vi "3001-CC.VI"() -> ()   [LabVIEW 2015]
uses:
  board.vis/Globals.vi
  <vilib>/Analysis/NI_AALBase.lvlib
panel:
  out "CAMCNT":dbl=2.0
  in  "extTrig":bool
  in  "ext. trig. slope":enum32{"1", "2", "3"}(radio)
  out "amount of devices":u8=1
  out "amount of cams":u8=2
  in  "CHB 8":bool
  in  "CHA 8":bool
  in  "CHB 7":bool
  in  "CHA 7":bool
  in  "CHB 6":bool
  in  "CHA 6":bool
  in  "CHB 5":bool
  in  "CHA 5":bool
  in  "CHB 4":bool
  in  "CHA 4":bool
  in  "CHB 3":bool
  in  "CHA 3":bool
  in  "CHB 2":bool
  in  "CHA 2":bool
  in  "CHB 1":bool=TRUE
  in  "CHA 1":bool=TRUE
  in  "channel quick select (in hex)":u16=3 format="%x"
  out "tRMS":dbl format="%0#.1f"
  out "mean":dbl format="%#_4f"
  in  "rms_pixel":u16=100
  in  "is FFT":bool=TRUE
  in  "IR gain":bool
  in  "continuous":bool=TRUE
  out "curr.block":u8=2
  out "Measure ON":bool
  in  "Board select\n1: board 1\n2: board 2\n3: both boards":u8=3
  in  "no.of blocks (nob)\npress enter":u32=1
  in  "block":u32(slide)=1 max=10 scale=0.9..1.0
  out "Signalverlaufgraph 2":u16[](graph)=[0, 0, 543, 543, 0, 1, 0, 0, 2, 2, 3, 3, 4, 4, 5, 5, 6, 6, 7, 7, 8, 8, 9, 9, 10, 10, 11, 11, 12, 12, 13, 13, 14, 14, 15, 15, 16, 16, 17, 17, 18, 18, 19, 19, 20, 20, 21, 21, 22, 22, 23, 23, 24, 24, 25, 25, 26, 26, 27, 27, 28, 28, 29, 29, 30, 30, 31, 31, 32, 32, 33, 33, 34, 34, 35, 35, 36, 36, 37, 37, 38, 38, 39, 39, 40, 40, 41, 41, 42, 42, 43, 43, 44, 44, 45, 45, 46, 46, 47, 47, 48, 48, 49, 49, 50, 50, 51, 51, 52, 52, 53, 53, 54, 54, 55, 55, 56, 56, 57, 57, 58, 58, 59, 59, 60, 60, 61, 61, 62, 62, 63, 63, 64, 64, 65, 65, 66, 66, 67, 67, 68, 68, 69, 69, 70, 70, 71, 71, 72, 72, 73, 73, 74, 74, 75, 75, 76, 76, 77, 77, 78, 78, 79, 79, 80, 80, 81, 81, 82, 82, 83, 83, 84, 84, 85, 85, 86, 86, 87, 87, 88, 88, 89, 89, 90, 90, 91, 91, 92, 92, 93, 93, 94, 94, 95, 95, 96, 96, 97, 97, 98, 98, 99, 99, 100, 100, 101, 101, 102, 102, 103, 103, 104, 104, 105, 105, 106, 106, 107, 107, 108, 108, 109, 109, 110, 110, 111, 111, 112, 112, 113, 113, 114, 114, 115, 115, 116, 116, 117, 117, 118, 118, 119, 119, 120, 120, 121, 121, 122, 122, 123, 123, 124, 124, 125, 125, 126, 126, 127, 127, 128, 128, 129, 129, 130, 130, 131, 131, 132, 132, 133, 133, 134, 134, 135, 135, 136, 136, 137, 137, 138, 138, 139, 139, 140, 140, 141, 141, 142, 142, 143, 143, 144, 144, 145, 145, 146, 146, 147, 147, 148, 148, 149, 149, 150, 150, 151, 151, 152, 152, 153, 153, 154, 154, 155, 155, 156, 156, 157, 157, 158, 158, 159, 159, 160, 160, 161, 161, 162, 162, 163, 163, 164, 164, 165, 165, 166, 166, 167, 167, 168, 168, 169, 169, 170, 170, 171, 171, 172, 172, 173, 173, 174, 174, 175, 175, 176, 176, 177, 177, 178, 178, 179, 179, 180, 180, 181, 181, 182, 182, 183, 183, 184, 184, 185, 185, 186, 186, 187, 187, 188, 188, 189, 189, 190, 190, 191, 191, 192, 192, 193, 193, 194, 194, 195, 195, 196, 196, 197, 197, 198, 198, 199, 199, 200, 200, 201, 201, 202, 202, 203, 203, 204, 204, 205, 205, 206, 206, 207, 207, 208, 208, 209, 209, 210, 210, 211, 211, 212, 212, 213, 213, 214, 214, 215, 215, 216, 216, 217, 217, 218, 218, 219, 219, 220, 220, 221, 221, 222, 222, 223, 223, 224, 224, 225, 225, 226, 226, 227, 227, 228, 228, 229, 229, 230, 230, 231, 231, 232, 232, 233, 233, 234, 234, 235, 235, 236, 236, 237, 237, 238, 238, 239, 239, 240, 240, 241, 241, 242, 242, 243, 243, 244, 244, 245, 245, 246, 246, 247, 247, 248, 248, 249, 249, 250, 250, 251, 251, 252, 252, 253, 253, 254, 254, 255, 255, 256, 256, 257, 257, 258, 258, 259, 259, 260, 260, 261, 261, 262, 262, 263, 263, 264, 264, 265, 265, 266, 266, 267, 267, 268, 268, 269, 269, 270, 270, 271, 271, 272, 272, 273, 273, 274, 274, 275, 275, 276, 276, 277, 277, 278, 278, 279, 279, 280, 280, 281, 281, 282, 282, 283, 283, 284, 284, 285, 285, 286, 286, 287, 287, 288, 288, 289, 289, 290, 290, 291, 291, 292, 292, 293, 293, 294, 294, 295, 295, 296, 296, 297, 297, 298, 298, 299, 299, 300, 300, 301, 301, 302, 302, 303, 303, 304, 304, 305, 305, 306, 306, 307, 307, 308, 308, 309, 309, 310, 310, 311, 311, 312, 312, 313, 313, 314, 314, 315, 315, 316, 316, 317, 317, 318, 318, 319, 319, 320, 320, 321, 321, 322, 322, 323, 323, 324, 324, 325, 325, 326, 326, 327, 327, 328, 328, 329, 329, 330, 330, 331, 331, 332, 332, 333, 333, 334, 334, 335, 335, 336, 336, 337, 337, 338, 338, 339, 339, 340, 340, 341, 341, 342, 342, 343, 343, 344, 344, 345, 345, 346, 346, 347, 347, 348, 348, 349, 349, 350, 350, 351, 351, 352, 352, 353, 353, 354, 354, 355, 355, 356, 356, 357, 357, 358, 358, 359, 359, 360, 360, 361, 361, 362, 362, 363, 363, 364, 364, 365, 365, 366, 366, 367, 367, 368, 368, 369, 369, 370, 370, 371, 371, 372, 372, 373, 373, 374, 374, 375, 375, 376, 376, 377, 377, 378, 378, 379, 379, 380, 380, 381, 381, 382, 382, 383, 383, 384, 384, 385, 385, 386, 386, 387, 387, 388, 388, 389, 389, 390, 390, 391, 391, 392, 392, 393, 393, 394, 394, 395, 395, 396, 396, 397, 397, 398, 398, 399, 399, 400, 400, 401, 401, 402, 402, 403, 403, 404, 404, 405, 405, 406, 406, 407, 407, 408, 408, 409, 409, 410, 410, 411, 411, 412, 412, 413, 413, 414, 414, 415, 415, 416, 416, 417, 417, 418, 418, 419, 419, 420, 420, 421, 421, 422, 422, 423, 423, 424, 424, 425, 425, 426, 426, 427, 427, 428, 428, 429, 429, 430, 430, 431, 431, 432, 432, 433, 433, 434, 434, 435, 435, 436, 436, 437, 437, 438, 438, 439, 439, 440, 440, 441, 441, 442, 442, 443, 443, 444, 444, 445, 445, 446, 446, 447, 447, 448, 448, 449, 449, 450, 450, 451, 451, 452, 452, 453, 453, 454, 454, 455, 455, 456, 456, 457, 457, 458, 458, 459, 459, 460, 460, 461, 461, 462, 462, 463, 463, 464, 464, 465, 465, 466, 466, 467, 467, 468, 468, 469, 469, 470, 470, 471, 471, 472, 472, 473, 473, 474, 474, 475, 475, 476, 476, 477, 477, 478, 478, 479, 479, 480, 480, 481, 481, 482, 482, 483, 483, 484, 484, 485, 485, 486, 486, 487, 487, 488, 488, 489, 489, 490, 490, 491, 491, 492, 492, 493, 493, 494, 494, 495, 495, 496, 496, 497, 497, 498, 498, 499, 499, 500, 500, 501, 501, 502, 502, 503, 503, 504, 504, 505, 505, 506, 506, 507, 507, 508, 508, 509, 509, 510, 510, 511, 511, 512, 512, 513, 513, 514, 514, 515, 515, 516, 516, 517, 517, 518, 518, 519, 519, 520, 520, 521, 521, 522, 522, 523, 523, 524, 524, 525, 525, 526, 526, 527, 527, 528, 528, 529, 529, 530, 530, 531, 531, 532, 532, 533, 533, 534, 534, 535, 535, 536, 536, 537, 537, 538, 538, 539, 539, 540, 540, 541, 541]
  out "Signalverlaufgraph":u16[](graph)=[544, 544, 545, 545, 49152, 1, 0, 0, 2, 2, 3, 3, 4, 4, 5, 5, 6, 6, 7, 7, 8, 8, 9, 9, 10, 10, 11, 11, 12, 12, 13, 13, 14, 14, 15, 15, 16, 16, 17, 17, 18, 18, 19, 19, 20, 20, 21, 21, 22, 22, 23, 23, 24, 24, 25, 25, 26, 26, 27, 27, 28, 28, 29, 29, 30, 30, 31, 31, 32, 32, 33, 33, 34, 34, 35, 35, 36, 36, 37, 37, 38, 38, 39, 39, 40, 40, 41, 41, 42, 42, 43, 43, 44, 44, 45, 45, 46, 46, 47, 47, 48, 48, 49, 49, 50, 50, 51, 51, 52, 52, 53, 53, 54, 54, 55, 55, 56, 56, 57, 57, 58, 58, 59, 59, 60, 60, 61, 61, 62, 62, 63, 63, 64, 64, 65, 65, 66, 66, 67, 67, 68, 68, 69, 69, 70, 70, 71, 71, 72, 72, 73, 73, 74, 74, 75, 75, 76, 76, 77, 77, 78, 78, 79, 79, 80, 80, 81, 81, 82, 82, 83, 83, 84, 84, 85, 85, 86, 86, 87, 87, 88, 88, 89, 89, 90, 90, 91, 91, 92, 92, 93, 93, 94, 94, 95, 95, 96, 96, 97, 97, 98, 98, 99, 99, 100, 100, 101, 101, 102, 102, 103, 103, 104, 104, 105, 105, 106, 106, 107, 107, 108, 108, 109, 109, 110, 110, 111, 111, 112, 112, 113, 113, 114, 114, 115, 115, 116, 116, 117, 117, 118, 118, 119, 119, 120, 120, 121, 121, 122, 122, 123, 123, 124, 124, 125, 125, 126, 126, 127, 127, 128, 128, 129, 129, 130, 130, 131, 131, 132, 132, 133, 133, 134, 134, 135, 135, 136, 136, 137, 137, 138, 138, 139, 139, 140, 140, 141, 141, 142, 142, 143, 143, 144, 144, 145, 145, 146, 146, 147, 147, 148, 148, 149, 149, 150, 150, 151, 151, 152, 152, 153, 153, 154, 154, 155, 155, 156, 156, 157, 157, 158, 158, 159, 159, 160, 160, 161, 161, 162, 162, 163, 163, 164, 164, 165, 165, 166, 166, 167, 167, 168, 168, 169, 169, 170, 170, 171, 171, 172, 172, 173, 173, 174, 174, 175, 175, 176, 176, 177, 177, 178, 178, 179, 179, 180, 180, 181, 181, 182, 182, 183, 183, 184, 184, 185, 185, 186, 186, 187, 187, 188, 188, 189, 189, 190, 190, 191, 191, 192, 192, 193, 193, 194, 194, 195, 195, 196, 196, 197, 197, 198, 198, 199, 199, 200, 200, 201, 201, 202, 202, 203, 203, 204, 204, 205, 205, 206, 206, 207, 207, 208, 208, 209, 209, 210, 210, 211, 211, 212, 212, 213, 213, 214, 214, 215, 215, 216, 216, 217, 217, 218, 218, 219, 219, 220, 220, 221, 221, 222, 222, 223, 223, 224, 224, 225, 225, 226, 226, 227, 227, 228, 228, 229, 229, 230, 230, 231, 231, 232, 232, 233, 233, 234, 234, 235, 235, 236, 236, 237, 237, 238, 238, 239, 239, 240, 240, 241, 241, 242, 242, 243, 243, 244, 244, 245, 245, 246, 246, 247, 247, 248, 248, 249, 249, 250, 250, 251, 251, 252, 252, 253, 253, 254, 254, 255, 255, 256, 256, 257, 257, 258, 258, 259, 259, 260, 260, 261, 261, 262, 262, 263, 263, 264, 264, 265, 265, 266, 266, 267, 267, 268, 268, 269, 269, 270, 270, 271, 271, 272, 272, 273, 273, 274, 274, 275, 275, 276, 276, 277, 277, 278, 278, 279, 279, 280, 280, 281, 281, 282, 282, 283, 283, 284, 284, 285, 285, 286, 286, 287, 287, 288, 288, 289, 289, 290, 290, 291, 291, 292, 292, 293, 293, 294, 294, 295, 295, 296, 296, 297, 297, 298, 298, 299, 299, 300, 300, 301, 301, 302, 302, 303, 303, 304, 304, 305, 305, 306, 306, 307, 307, 308, 308, 309, 309, 310, 310, 311, 311, 312, 312, 313, 313, 314, 314, 315, 315, 316, 316, 317, 317, 318, 318, 319, 319, 320, 320, 321, 321, 322, 322, 323, 323, 324, 324, 325, 325, 326, 326, 327, 327, 328, 328, 329, 329, 330, 330, 331, 331, 332, 332, 333, 333, 334, 334, 335, 335, 336, 336, 337, 337, 338, 338, 339, 339, 340, 340, 341, 341, 342, 342, 343, 343, 344, 344, 345, 345, 346, 346, 347, 347, 348, 348, 349, 349, 350, 350, 351, 351, 352, 352, 353, 353, 354, 354, 355, 355, 356, 356, 357, 357, 358, 358, 359, 359, 360, 360, 361, 361, 362, 362, 363, 363, 364, 364, 365, 365, 366, 366, 367, 367, 368, 368, 369, 369, 370, 370, 371, 371, 372, 372, 373, 373, 374, 374, 375, 375, 376, 376, 377, 377, 378, 378, 379, 379, 380, 380, 381, 381, 382, 382, 383, 383, 384, 384, 385, 385, 386, 386, 387, 387, 388, 388, 389, 389, 390, 390, 391, 391, 392, 392, 393, 393, 394, 394, 395, 395, 396, 396, 397, 397, 398, 398, 399, 399, 400, 400, 401, 401, 402, 402, 403, 403, 404, 404, 405, 405, 406, 406, 407, 407, 408, 408, 409, 409, 410, 410, 411, 411, 412, 412, 413, 413, 414, 414, 415, 415, 416, 416, 417, 417, 418, 418, 419, 419, 420, 420, 421, 421, 422, 422, 423, 423, 424, 424, 425, 425, 426, 426, 427, 427, 428, 428, 429, 429, 430, 430, 431, 431, 432, 432, 433, 433, 434, 434, 435, 435, 436, 436, 437, 437, 438, 438, 439, 439, 440, 440, 441, 441, 442, 442, 443, 443, 444, 444, 445, 445, 446, 446, 447, 447, 448, 448, 449, 449, 450, 450, 451, 451, 452, 452, 453, 453, 454, 454, 455, 455, 456, 456, 457, 457, 458, 458, 459, 459, 460, 460, 461, 461, 462, 462, 463, 463, 464, 464, 465, 465, 466, 466, 467, 467, 468, 468, 469, 469, 470, 470, 471, 471, 472, 472, 473, 473, 474, 474, 475, 475, 476, 476, 477, 477, 478, 478, 479, 479, 480, 480, 481, 481, 482, 482, 483, 483, 484, 484, 485, 485, 486, 486, 487, 487, 488, 488, 489, 489, 490, 490, 491, 491, 492, 492, 493, 493, 494, 494, 495, 495, 496, 496, 497, 497, 498, 498, 499, 499, 500, 500, 501, 501, 502, 502, 503, 503, 504, 504, 505, 505, 506, 506, 507, 507, 508, 508, 509, 509, 510, 510, 511, 511, 512, 512, 513, 513, 514, 514, 515, 515, 516, 516, 517, 517, 518, 518, 519, 519, 520, 520, 521, 521, 522, 522, 523, 523, 524, 524, 525, 525, 526, 526, 527, 527, 528, 528, 529, 529, 530, 530, 531, 531, 532, 532, 533, 533, 534, 534, 535, 535, 536, 536, 537, 537, 538, 538, 539, 539, 540, 540, 541, 541]
  out "boards recognised":u8=1
  in  "alloc mem":bool
  out "FREE \nRAM MB":dbl=14650.41015625
  out "BUILT-IN\nRAM MB":dbl=18096.171875
  out "SEC":dbl=0.1
  out "MB RAM":dbl=0.4150390625
  in  "DAT in 10ns":u32
  in  "stop all":bool
  in  "start":bool
  in  "sample":u32(slide)=974 max=3000 scale=0.9..100.0
  in  "no.of samples (nos)":u32=100
  in  "exposuretime[ms]":dbl=1.0 format="%.3f"
  # "Camera Control 1"
  # "Camera Control 5"
  # "Camera Control 2"
  # "Camera Control 6"
  # "Camera Control 3"
  # "Camera Control 7"
  # "Camera Control 4"
  # "Camera Control 8"
  # "press Esc to stop measurement"
  # "exit here"
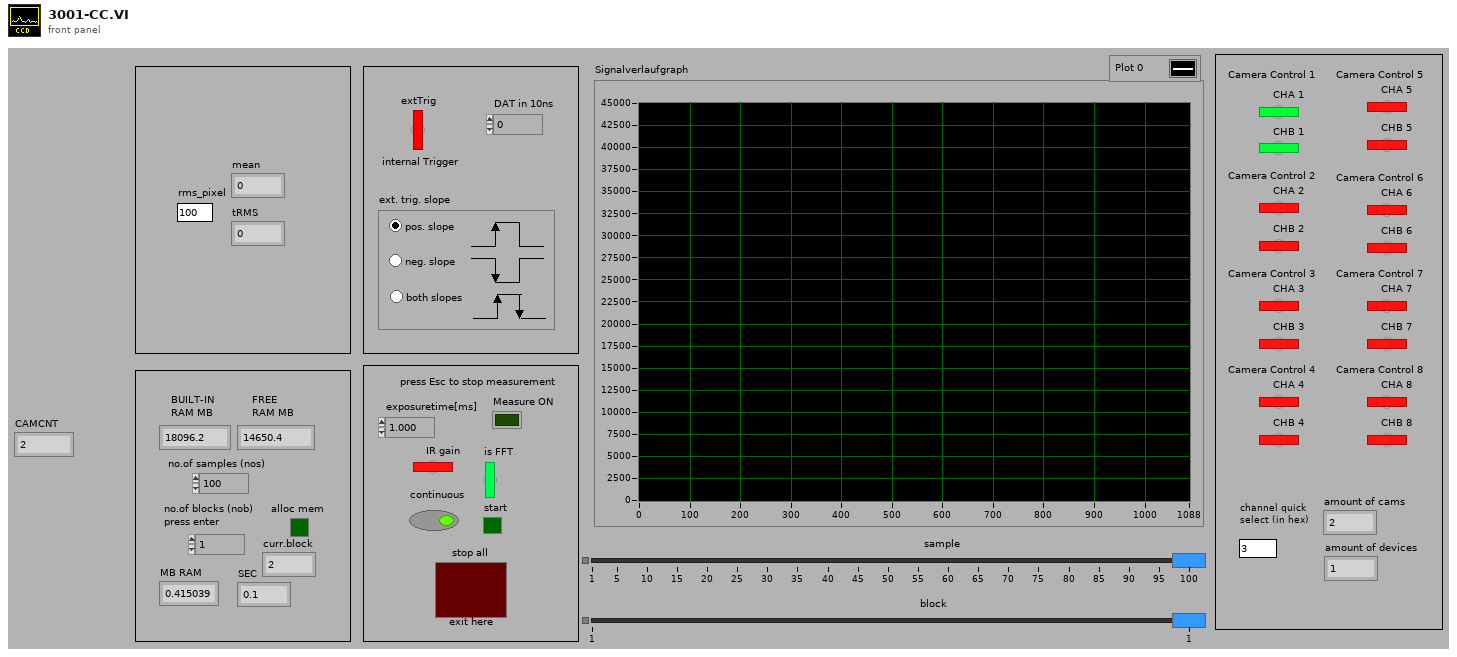
[diagram p1: front panel]
types:
  T1 = enum8{"Enabled", "Disabled", "Disabled and Grayed Out"}
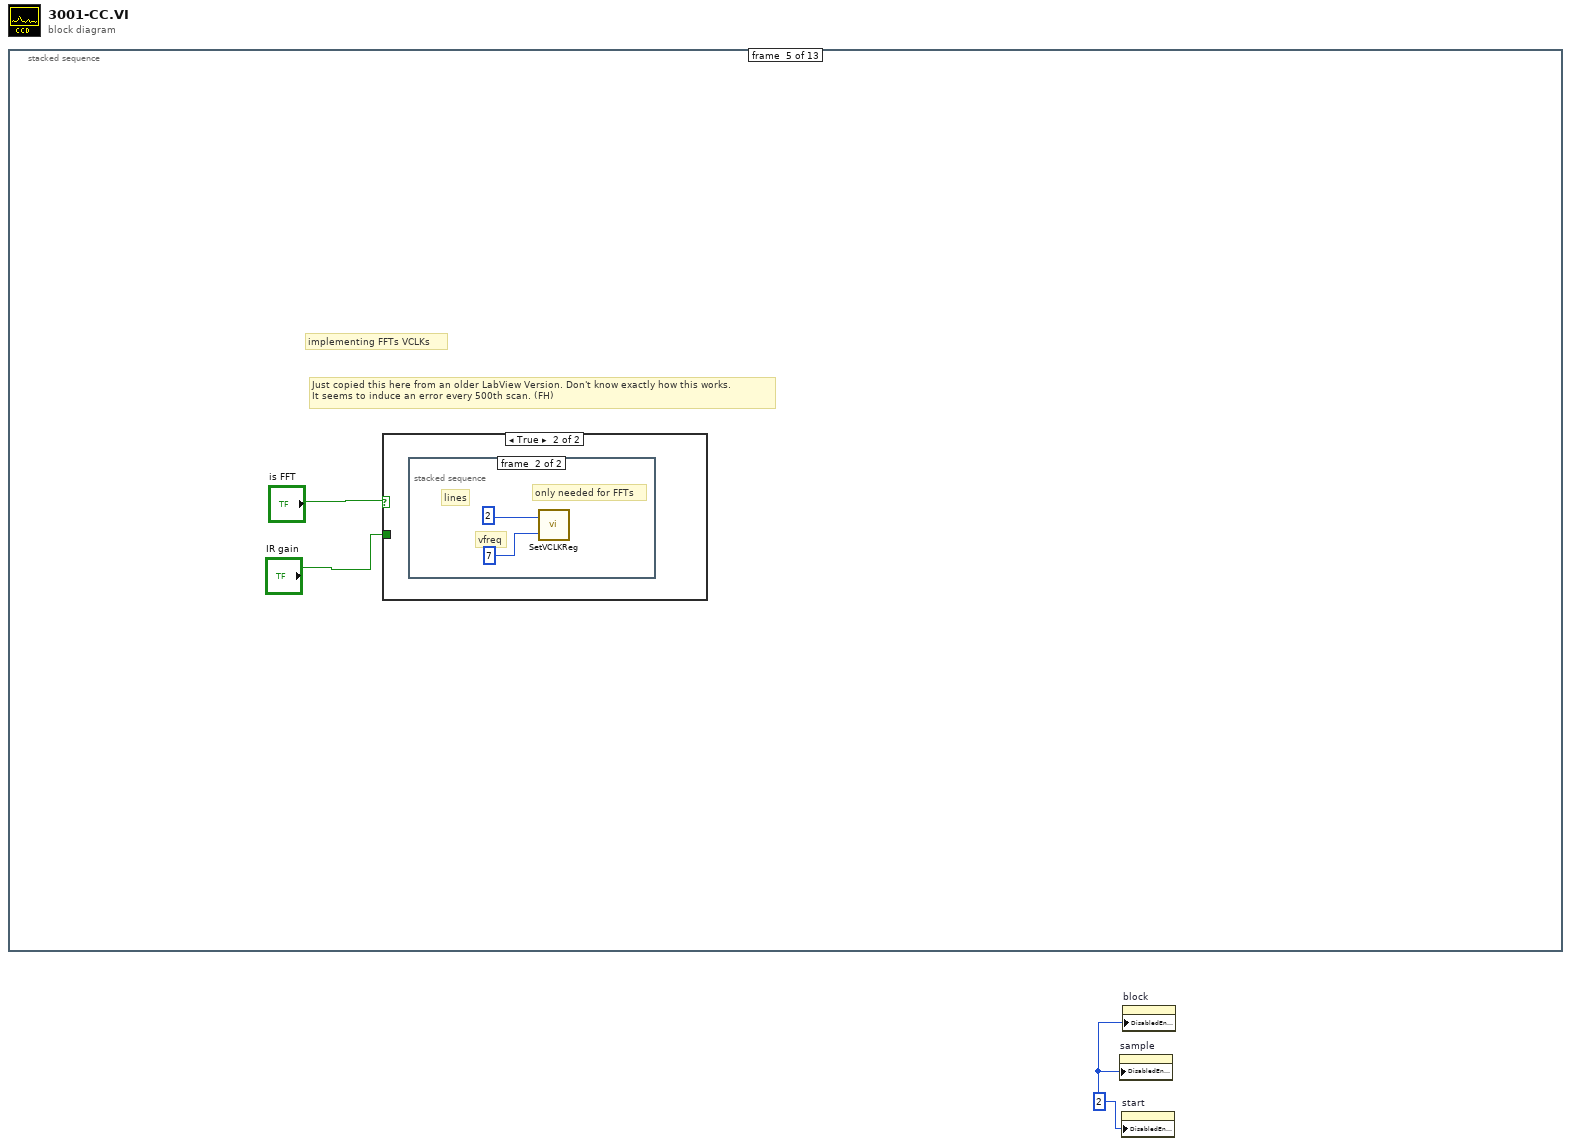
[diagram p0: block diagram]
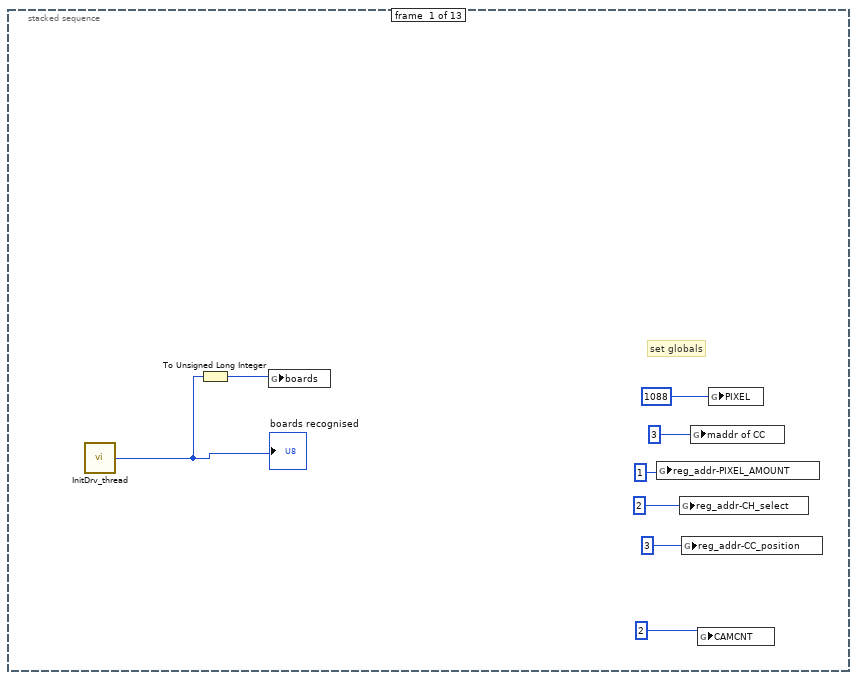
[diagram p2: hidden frame]
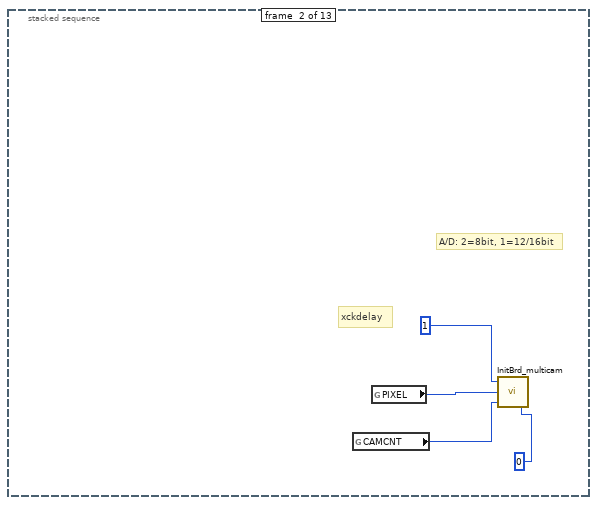
[diagram p3: hidden frame]
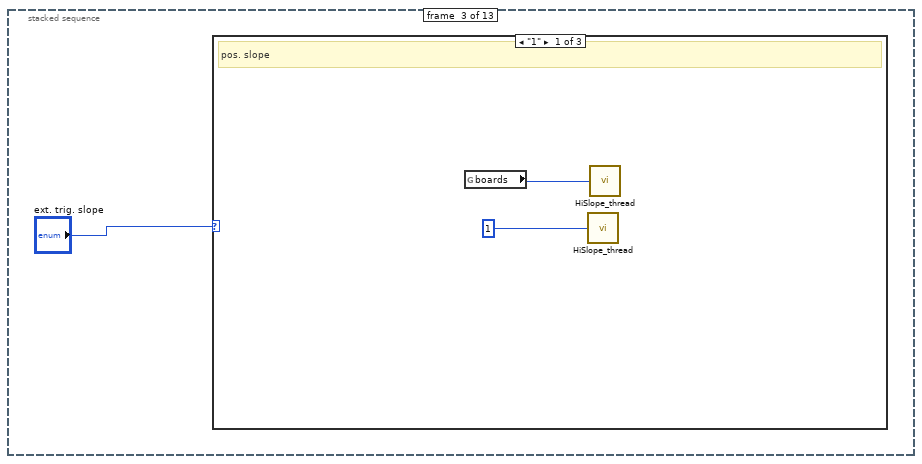
[diagram p4: hidden frame]
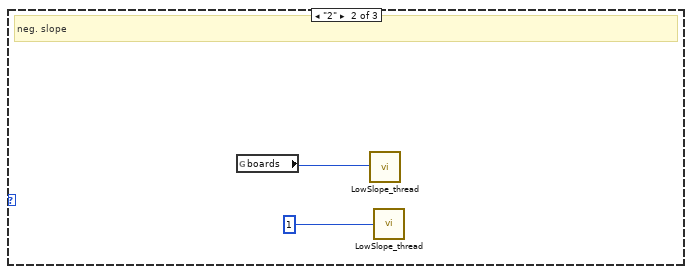
[diagram p5: hidden frame]
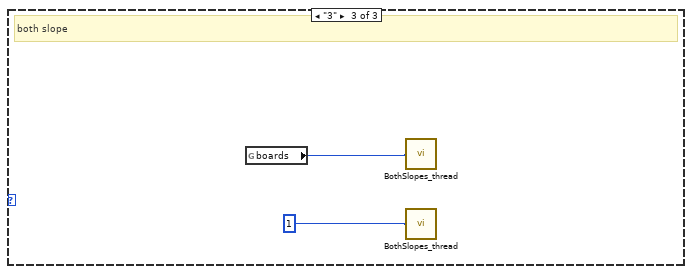
[diagram p6: hidden frame]
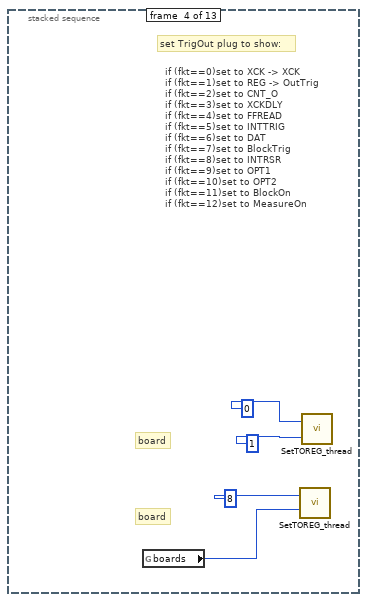
[diagram p7: hidden frame]
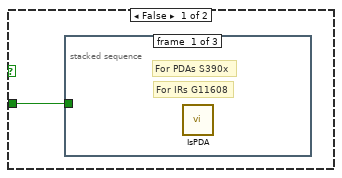
[diagram p8: hidden frame]
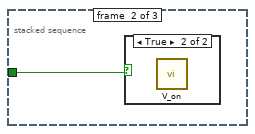
[diagram p9: hidden frame]
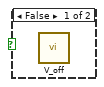
[diagram p10: hidden frame]
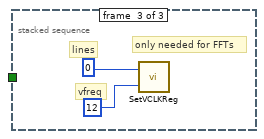
[diagram p11: hidden frame]
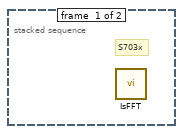
[diagram p12: hidden frame]
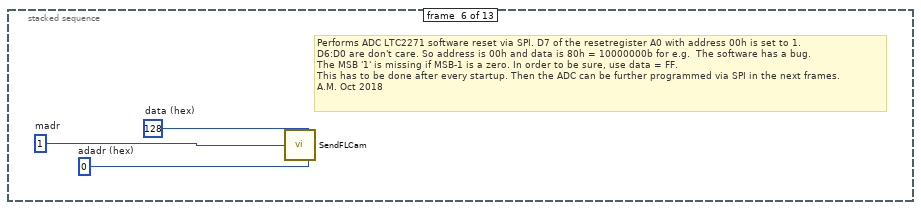
[diagram p13: hidden frame]
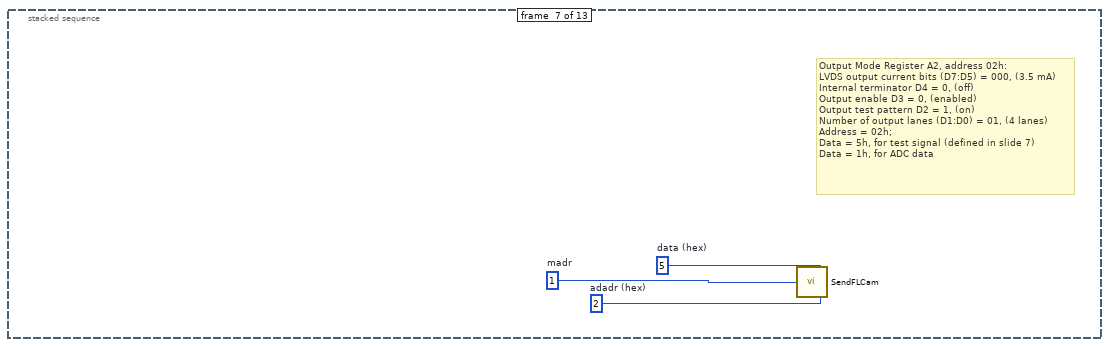
[diagram p14: hidden frame]
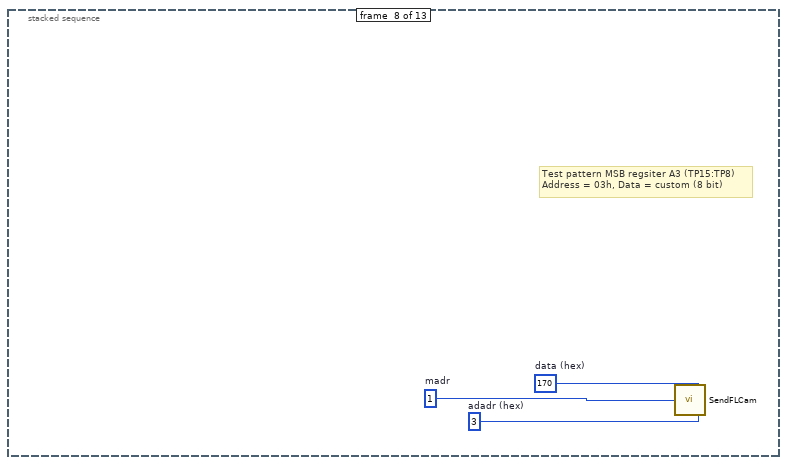
[diagram p15: hidden frame]
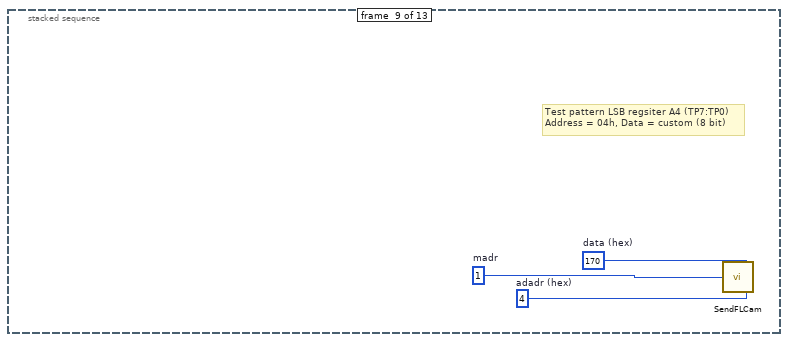
[diagram p16: hidden frame]
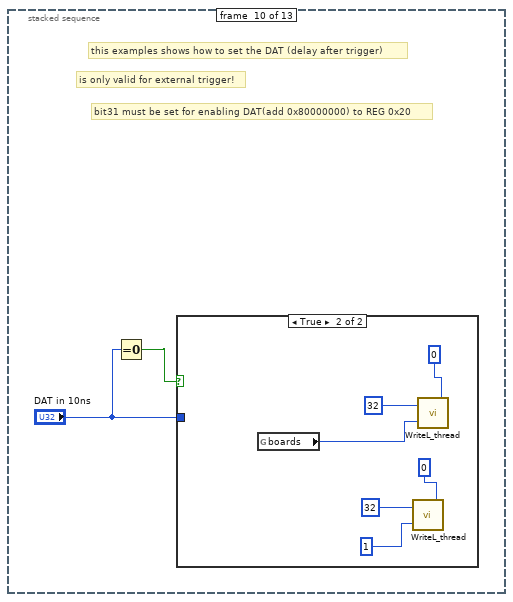
[diagram p17: hidden frame]
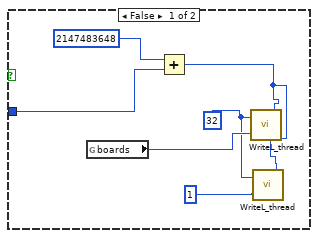
[diagram p18: hidden frame]
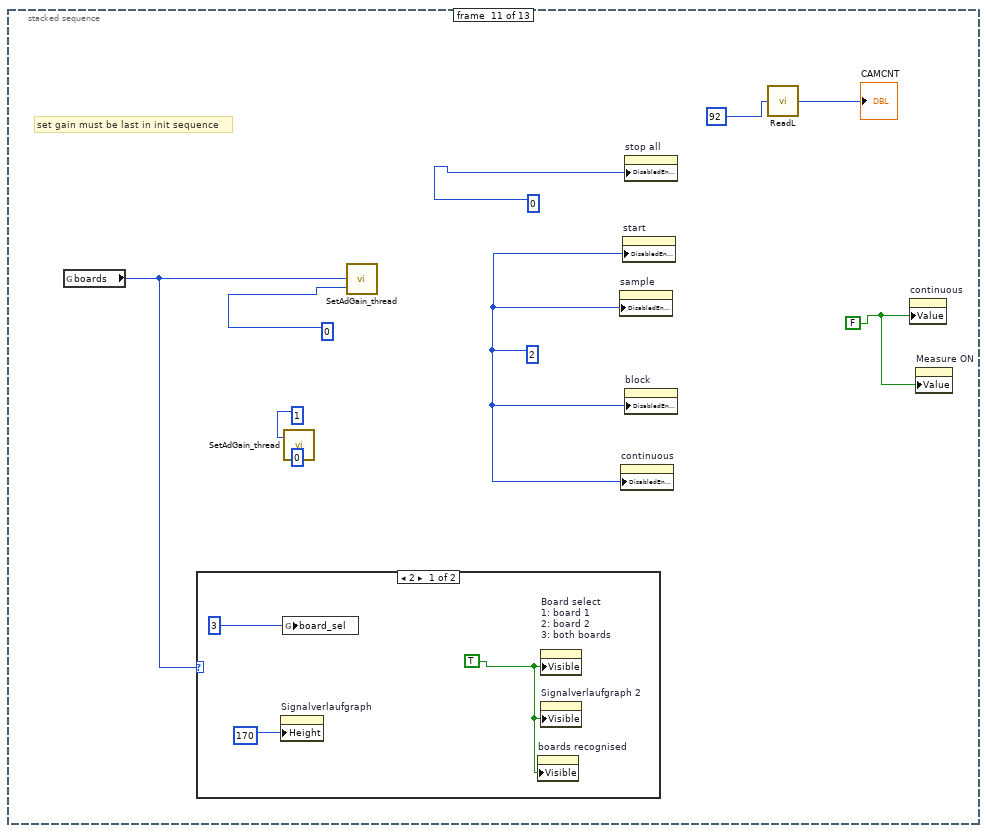
[diagram p19: hidden frame]
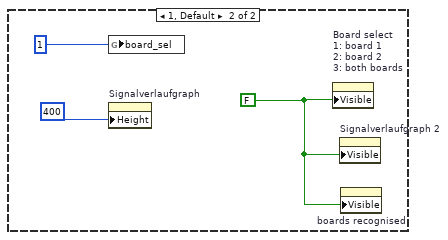
[diagram p20: hidden frame]
diagram:
  w1 = 2
  n1 = stacked-sequence {
    frame #0 {
      # "set globals"
      n2 = call "InitDrv_thread.vi"() -> ("Boards"=w7:u8)  [unwired: 1 in]
      "boards recognised" <- w7
      n3 = To Unsigned Long Integer(number=w7) -> (unsigned 32bit integer=w8:u32)
      n4 = global write "Globals.vi" "boards"(w8) -> ()
      n5 = global write "Globals.vi" "reg_addr-PIXEL_AMOUNT"(u8 1) -> ()
      n6 = global write "Globals.vi" "reg_addr-CH_select"(u8 2) -> ()
      n7 = global write "Globals.vi" "reg_addr-CC_position"(u8 3) -> ()
      n8 = global write "Globals.vi" "maddr of CC"(u8 3) -> ()
      n9 = global write "Globals.vi" "CAMCNT"(u32 2) -> ()
      n10 = global write "Globals.vi" "PIXEL"(u32 1088) -> ()
    }
    frame #1 {
      # "xckdelay"
      # "A/D: 2=8bit, 1=12/16bit"
      n11 = global read "Globals.vi" "CAMCNT"() -> (w10:u32)
      n12 = global read "Globals.vi" "PIXEL"() -> (w13:u32)
      n13 = call "InitBrd_multicam.vi"("xckdly"=u32 0, "camcnt"=w10, "pixel"=w13, "flag816"=u32 1) -> ()  [unwired: 2 in]
    }
    frame #2 {
      n14 = case shown="\"1\"" "ext. trig. slope" {
        frame "1" {
          # "pos. slope"
          n15 = global read "Globals.vi" "boards"() -> (w15:u32)
          n16 = call "HiSlope_thread.vi"("board"=u32 1) -> ()  [unwired: 1 in]
          n17 = call "HiSlope_thread.vi"("board"=w15) -> ()  [unwired: 1 in]
        }
        frame "2" {
          # "neg. slope"
          n18 = global read "Globals.vi" "boards"() -> (w18:u32)
          n19 = call "LowSlope_thread.vi"("board"=w18) -> ()  [unwired: 1 in]
          n20 = call "LowSlope_thread.vi"("board"=u32 1) -> ()  [unwired: 1 in]
        }
        frame "3" {
          # "both slope"
          n21 = global read "Globals.vi" "boards"() -> (w19:u32)
          n22 = call "BothSlopes_thread.vi"("board"=w19) -> ()  [unwired: 1 in]
          n23 = call "BothSlopes_thread.vi"("board"=u32 1) -> ()  [unwired: 1 in]
        }
      }
    }
    frame #3 {
      # "board"
      # "board"
      # "set TrigOut plug to show:"
      # "if (fkt==0)set to XCK -> XCK\nif (fkt==1)set to REG -> OutTrig\nif (fkt==2)set to CNT_O\nif (fkt==3)set to XCKDLY\nif (fkt==4)set to FFREAD\nif (fkt==5)set to INTTRIG\nif (fkt==6)set to DAT\nif (fkt==7)set to BlockTrig\nif (fkt==8)set to INTRSR\nif (fkt==9)set to OPT1\nif (fkt==10)set to OPT2\nif (fkt==11)set to BlockOn\nif (fkt==12)set to MeasureOn"
      n24 = global read "Globals.vi" "boards"() -> (w24:u32)
      n25 = call "SetTOREG_thread.vi"("board"=w24, "fkt"=u8 8) -> ()  [unwired: 1 in]
      n26 = call "SetTOREG_thread.vi"("board"=u32 1, "fkt"=u8 0) -> ()  [unwired: 1 in]
    }
    frame #4 {
      # "implementing FFTs VCLKs"
      # "Just copied this here from an older LabView Version. Don't know exactly how this works.\nIt seems to induce an error every 500th scan. (FH)"
      n27 = case shown="True" "is FFT" {
        tunnel: "IR gain" -> [w27 _]
        frame False {
          n28 = stacked-sequence {
            tunnel: w27 -> [_ w28 _]
            frame #0 {
              # "For IRs G11608"
              # "For PDAs S390x"
              n29 = call "IsPDA.vi"() -> ()  [unwired: 1 in]
            }
            frame #1 {
              n30 = case shown="True" w28 {
                frame False {
                  n31 = call "V_off.vi"() -> ()  [unwired: 1 in]
                }
                frame True {
                  n32 = call "V_on.vi"() -> ()  [unwired: 1 in]
                }
              }
            }
            frame #2 {
              # "only needed for FFTs"
              # "vfreq"
              # "lines"
              n33 = call "SetVCLKReg.vi"("vfreq"=u8 12, "lines"=u32 0) -> ()  [unwired: 1 in]
            }
          }
        }
        frame True {
          n34 = stacked-sequence {
            frame #0 {
              # "S703x"
              n35 = call "IsFFT.vi"() -> ()  [unwired: 1 in]
            }
            frame #1 {
              # "only needed for FFTs"
              # "vfreq"
              # "lines"
              n36 = call "SetVCLKReg.vi"("vfreq"=u8 7, "lines"=u32 2) -> ()  [unwired: 1 in]
            }
          }
        }
      }
    }
    frame #5 {
      w33 = u16 128  # data (hex)
      w34 = u8 0  # adadr (hex)
      w35 = u8 1  # madr
      # "Performs ADC LTC2271 software reset via SPI. D7 of the resetregister A0 with address 00h is set to 1.\nD6:D0 are don't care. So address is 00h and data is 80h = 10000000b for e.g.  The software has a bug.\nThe MSB '1' is missing if MSB-1 is a zero. In order to be sure, use data = FF.\nThis has to be done after every startup. Then the ADC can be further programmed via SPI in the next frames.\nA.M. Oct 2018"
      n37 = call "SendFLCam.vi"("madr"=w35, "data"=w33, "adadr"=w34) -> ()
    }
    frame #6 {
      w36 = u16 5  # data (hex)
      w37 = u8 2  # adadr (hex)
      w38 = u8 1  # madr
      # "Output Mode Register A2, address 02h:\nLVDS output current bits (D7:D5) = 000, (3.5 mA)\nInternal terminator D4 = 0, (off)\nOutput enable D3 = 0, (enabled)\nOutput test pattern D2 = 1, (on)\nNumber of output lanes (D1:D0) = 01, (4 lanes)\nAddress = 02h;\nData = 5h, for test signal (defined in slide 7)\nData = 1h, for ADC data"
      n38 = call "SendFLCam.vi"("madr"=w38, "data"=w36, "adadr"=w37) -> ()
    }
    frame #7 {
      w39 = u16 170  # data (hex)
      w40 = u8 3  # adadr (hex)
      w41 = u8 1  # madr
      # "Test pattern MSB regsiter A3 (TP15:TP8)\nAddress = 03h, Data = custom (8 bit)"
      n39 = call "SendFLCam.vi"("madr"=w41, "data"=w39, "adadr"=w40) -> ()
    }
    frame #8 {
      w42 = u16 170  # data (hex)
      w43 = u8 4  # adadr (hex)
      w44 = u8 1  # madr
      # "Test pattern LSB regsiter A4 (TP7:TP0)\nAddress = 04h, Data = custom (8 bit)"
      n40 = call "SendFLCam.vi"("madr"=w44, "data"=w42, "adadr"=w43) -> ()
    }
    frame #9 {
      # "bit31 must be set for enabling DAT(add 0x80000000) to REG 0x20"
      # "is only valid for external trigger!"
      # "this examples shows how to set the DAT (delay after trigger)"
      n41 = Equal To 0?(x="DAT in 10ns") -> (x = 0?=w46:bool)
      n42 = case shown="True" w46 {
        tunnel: "DAT in 10ns" -> [w51 _]
        frame False {
          w48 = u32 32
          n43 = global read "Globals.vi" "boards"() -> (w50:u32)
          n44 = Add(x=u32 2147483648, y=w51) -> (x+y=w49:u32)
          n45 = call "WriteL_thread.vi"("val"=w49, "board"=w50, "offset"=w48) -> ()
          n46 = call "WriteL_thread.vi"("val"=w49, "board"=u32 1, "offset"=w48) -> ()
        }
        frame True {
          n47 = global read "Globals.vi" "boards"() -> (w57:u32)
          n48 = call "WriteL_thread.vi"("val"=u32 0, "board"=u32 1, "offset"=u32 32) -> ()
          n49 = call "WriteL_thread.vi"("val"=u32 0, "board"=w57, "offset"=u32 32) -> ()
        }
      }
    }
    frame #10 {
      w61 = FALSE
      w67 = 2
      # "set gain must be last in init sequence"
      n50 = global read "Globals.vi" "boards"() -> (w65:u32)
      n51 = case shown="2" w65 {
        frame 2 {
          w70 = TRUE
          n52 = property on="Signalverlaufgraph" class="WFGraph (strict)"("Height"=u8 170) -> ()  [unwired: 2 in, 2 out]
          n53 = global write "Globals.vi" "board_sel"(u8 3) -> ()
          n54 = property on="boards recognised" class="DigNum (strict)"("Visible"=w70) -> ()  [unwired: 2 in, 2 out]
          n55 = property on="Board select\n1: board 1\n2: board 2\n3: both boards" class="DigNum (strict)"("Visible"=w70) -> ()  [unwired: 2 in, 2 out]
          n56 = property on="Signalverlaufgraph 2" class="WFGraph (strict)"("Visible"=w70) -> ()  [unwired: 2 in, 2 out]
        }
        frame 1, Default {
          w71 = FALSE
          n57 = global write "Globals.vi" "board_sel"(u8 1) -> ()
          n58 = property on="Signalverlaufgraph" class="WFGraph (strict)"("Height"=400) -> ()  [unwired: 2 in, 2 out]
          n59 = property on="Board select\n1: board 1\n2: board 2\n3: both boards" class="DigNum (strict)"("Visible"=w71) -> ()  [unwired: 2 in, 2 out]
          n60 = property on="Signalverlaufgraph 2" class="WFGraph (strict)"("Visible"=w71) -> ()  [unwired: 2 in, 2 out]
          n61 = property on="boards recognised" class="DigNum (strict)"("Visible"=w71) -> ()  [unwired: 2 in, 2 out]
        }
      }
      n62 = call "SetAdGain_thread.vi"("gain"=u8 0, "board"=u32 1) -> ()  [unwired: 1 in]
      n63 = call "SetAdGain_thread.vi"("gain"=u8 0, "board"=w65) -> ()  [unwired: 1 in]
      n64 = property on="sample" class="Slide (strict)"("DisabledEnum"=w67) -> ()  [unwired: 2 in, 2 out]
      n65 = property on="continuous" class="Bool (strict)"("DisabledEnum"=w67) -> ()  [unwired: 2 in, 2 out]
      n66 = property on="start" class="Bool (strict)"("DisabledEnum"=w67) -> ()  [unwired: 2 in, 2 out]
      n67 = property on="stop all" class="Bool (strict)"("DisabledEnum"=0) -> ()  [unwired: 2 in, 2 out]
      n68 = property on="block" class="Slide (strict)"("DisabledEnum"=w67) -> ()  [unwired: 2 in, 2 out]
      n69 = call "ReadL.vi"("Offset"=u32 92) -> ("Data"=→"CAMCNT":u32)
      n70 = property on="continuous" class="Bool (strict)"("Value"=w61) -> ()  [unwired: 2 in, 2 out]
      n71 = property on="Measure ON" class="Bool (strict)"("Value"=w61) -> ()  [unwired: 2 in, 2 out]
    }
    frame #11 {
      # "Init Sequenz of Camera Control"
      n72 = flat-sequence {
        frame #0 {
          # "pixel_für_aurora in cam_control_gerät"
          n73 = global read "Globals.vi" "PIXEL"() -> (w75:u32)
          n74 = global read "Globals.vi" "reg_addr-PIXEL_AMOUNT"() -> (w79:u8)
          n75 = global read "Globals.vi" "maddr of CC"() -> (w78:u8)
          n76 = Multiply(x=w75, y=1) -> (x*y=w76:u32)
          n77 = To Unsigned Word Integer(number=w76) -> (unsigned 16bit integer=w77:u16)
          n78 = call "SendFLCam.vi"("madr"=w78, "data"=w77, "adadr"=w79) -> ()
        }
        frame #1 {
          n79 = global read "Globals.vi" "maddr of CC"() -> (w82:u8)
          n80 = global read "Globals.vi" "reg_addr-CH_select"() -> (w81:u8)
          n81 = property on="channel quick select (in hex)" class="DigNum (strict)"() -> ("Value"=w80:u16)  [unwired: 2 in, 2 out]
          n82 = call "SendFLCam.vi"("madr"=w82, "data"=w80, "adadr"=w81) -> ()
        }
        frame #2 {
          n83 = global read "Globals.vi" "maddr of CC"() -> (w85:u8)
          n84 = global read "Globals.vi" "reg_addr-CC_position"() -> (w84:u8)
          n85 = call "SendFLCam.vi"("madr"=w85, "data"=u16 1, "adadr"=w84) -> ()
        }
      }
    }
    frame #12 {
      n86 = while {
        stop <- w87 stop-if-true
        n87 = event shown="[6] \"sample\", \"block\": Value Change" {
          selector: _ -> [_ _ _ _ _ _ _ _ _ _ _ _]
          dyn-events: _ -> [_ _ _ _ _ _ _ _ _ _ _ _]
          timeout: 100 -> [_ _ _ _ _ _ _ _ _ _ _ _]
          tunnel: [_ _ _ _ _ _ _ _ _ _ w339 _] -> w87
          event Timeout {
            # "only refresh the frames if measure on"
            # "compares measure on signal from hardware with measure on lamp\nwhen diffrent than write new measure on value to lamp"
            # "timout excecutes every 100ms"
            # "userinfo of RAM, MeasureOB, Curr.Block and setting display event in cont mode"
            n88 = event-data() -> ()  [unwired: 1 in, 3 out]
            n89 = call "ReadB.vi"("Offset"=u32 64) -> ("Data"=w102:u8)
            n90 = call "FreeMemInfo.vi"() -> ("PhysicalSpace"=→"BUILT-IN\nRAM MB":dbl, "PhysicalFreeSpace"=→"FREE \nRAM MB":dbl)  [unwired: 1 in]
            n91 = Number To Boolean Array(number=w102) -> (Boolean array=w101:bool[])
            n92 = property on="Measure ON" class="Bool (strict)"() -> ("Value"=w95:bool)  [unwired: 2 in, 2 out]
            n93 = Index Array(array=w101, index=5) -> (element=w91:bool)
            n94 = Not Equal?(x=w95, y=w91) -> (x != y?=w94:bool)
            n95 = case shown="True" w94 {
              tunnel: w91 -> [_ w106]
              frame False {
              }
              frame True {
                n96 = property on="Measure ON" class="Bool (strict)"("Val(Sgnl)"=w106) -> ()  [unwired: 2 in, 2 out]
              }
            }
            n97 = property on="continuous" class="Bool (strict)"() -> ("DisabledEnum"=w88:T1)  [unwired: 2 in, 2 out]
            n98 = property on="continuous" class="Bool (strict)"() -> ("Value"=w97:bool)  [unwired: 2 in, 2 out]
            n99 = To Unsigned Byte Integer(number=w88) -> (unsigned 8bit integer=w89:u8)
            n100 = Equal?(x=w89, y=u8 0) -> (x = y?=w96:bool)
            n101 = And(x=w97, y=w96) -> (x .and. y?=w93:bool)
            n102 = And(x=w93, y=w91) -> (x .and. y?=w92:bool)
            n103 = call "ReadB.vi"("Offset"=u32 88) -> ("Data"=→"curr.block":u8)
            n104 = case shown="True" w92 {
              frame False {
              }
              frame True {
                # "refresh RMS.\nMaybe this is not a good style.\nIt's not clear to me which values are \nincluded to RMS measurement.\nBetter would be a refresh when all\nblocks are done."
                # "trigger the \ndisplay event"
                n105 = property on="rms_pixel" class="DigNum (strict)"() -> ("Value"=w107:u16)  [unwired: 2 in, 2 out]
                n106 = property on="sample" class="Slide (strict)"() -> ("Value"=w108:u32)  [unwired: 2 in, 2 out]
                n107 = property on="sample" class="Slide (strict)"("Val(Sgnl)"=w108) -> ()  [unwired: 2 in, 2 out]
                n108 = property on="rms_pixel" class="DigNum (strict)"("Val(Sgnl)"=w107) -> ()  [unwired: 2 in, 2 out]
              }
            }
          }
          event "Measure ON": Value Change {
            # "triggers on value change of measure on. this happens on start of measurement and after measurement\nwhen continuous: not after finishing all blocks, only when exiting measurement"
            n109 = event-data() -> ("NewVal"=w109:bool)  [unwired: 1 in, 5 out]
            n110 = property on="continuous" class="Bool (strict)"() -> ("Value"=w110:bool)  [unwired: 2 in, 2 out]
            n111 = And(x=w110, y=w109) -> (x .and. y?=w111:bool)
            n112 = case shown="False" w109 {
              frame False {
                n113 = property on="stop all" class="Bool (strict)"("DisabledEnum"=0) -> ()  [unwired: 2 in, 2 out]
              }
              frame True {
              }
            }
            n114 = case shown="True" w111 {
              frame False {
              }
              frame True {
                n115 = property on="stop all" class="Bool (strict)"("DisabledEnum"=2) -> ()  [unwired: 2 in, 2 out]
              }
            }
          }
          event "Board select\n1: board 1\n2: board 2\n3: both boards": Value Change {
            # "selecting number of cams"
            n116 = event-data() -> ()  [unwired: 1 in, 6 out]
            n117 = global read "Globals.vi" "boards"() -> (w114:u32)
            n118 = case shown="2" w114 {
              frame 0, Default {
              }
              frame 2 {
                n119 = global write "Globals.vi" "board_sel"("Board select\n1: board 1\n2: board 2\n3: both boards") -> ()
              }
            }
          }
          event "continuous": Value Change {
            # "setting continuos mode"
            n120 = event-data() -> ()  [unwired: 1 in, 6 out]
            n121 = case shown="False" "continuous" {
              tunnel: [u8 0 u8 1] -> w116
              frame False {
              }
              frame True {
              }
            }
            n122 = call "contFFLoop.vi"("Numeric"=w116) -> ()  [unwired: 1 in]
          }
          event "alloc mem": Value Change {
            w126 = 0
            # "update params"
            # "Setup DMA"
            n123 = event-data() -> ()  [unwired: 1 in, 6 out]
            n124 = global read "Globals.vi" "cams_amount"() -> (w123:u8)
            n125 = global read "Globals.vi" "nob"() -> (w124:u32)
            n126 = global read "Globals.vi" "nos"() -> (w125:u32)
            n127 = To Unsigned Long Integer(number=w123) -> (unsigned 32bit integer=w122:u32)
            n128 = global read "Globals.vi" "boards"() -> (w129:u32)
            n129 = Multiply(x=w122, y=w124) -> (x*y=w120:u32)
            n130 = Multiply(x=w122, y=w125) -> (x*y=w121:u32)
            n131 = case shown="2" w129 {
              selector: w129 -> [_ w130]
              tunnel: w121 -> [_ w131]
              tunnel: w120 -> [_ w132]
              frame 1, Default {
              }
              frame 2 {
                # "Setup DMA"
                n132 = call "SetupDMA_thread.vi"("blocks"=w132, "nos"=w131, "Drv"=w130) -> ()  [unwired: 2 in]
              }
            }
            n133 = call "SetupDMA_thread.vi"("blocks"=w120, "nos"=w121, "Drv"=u32 1) -> ()  [unwired: 2 in]
            n134 = property on="continuous" class="Bool (strict)"("DisabledEnum"=w126) -> ()  [unwired: 2 in, 2 out]
            n135 = property on="block" class="Slide (strict)"("DisabledEnum"=w126) -> ()  [unwired: 2 in, 2 out]
            n136 = property on="sample" class="Slide (strict)"("DisabledEnum"=w126) -> ()  [unwired: 2 in, 2 out]
            n137 = property on="exposuretime[ms]" class="DigNum (strict)"() -> ("Value"=w128:dbl)  [unwired: 2 in, 2 out]
            n138 = property on="start" class="Bool (strict)"("DisabledEnum"=w126) -> ()  [unwired: 2 in, 2 out]
            n139 = property on="exposuretime[ms]" class="DigNum (strict)"("Val(Sgnl)"=w128) -> ()  [unwired: 2 in, 2 out]
          }
          event "start": Mouse Down {
            # "start measurement"
            # "only 1st PCI board is used for ext. trig."
            # "ext. block trig\n0: internal: Space\n1: PCI \"I\"\n2: S1\n3: S2"
            # "block trigger 0/1\n0: internal -> next block is started immediately \n1: external -> each block has an own trigger"
            n140 = event-data() -> ()  [unwired: 1 in, 8 out]
            n141 = global read "Globals.vi" "exp time"() -> (w139:dbl)
            n142 = Multiply(x=1000.0, y=w139) -> (x*y=w141:dbl)
            n143 = global read "Globals.vi" "board_sel"() -> (w135:u8)
            n144 = To Unsigned Long Integer(number=w141) -> (unsigned 32bit integer=w137:u32)
            n145 = case shown="True" "extTrig" {
              tunnel: [u8 0 u8 1] -> w134
              frame False {
              }
              frame True {
              }
            }
            n146 = call "ReadFFLoop_thread.vi"("blocktrigger"=u8 0, "btrig_ch"=u8 0, "ExtTrig"=w134, "cam_sel"=w135, "exptus"=w137) -> ()  [unwired: 1 in]
          }
          event "sample", "block": Value Change {
            w155 = u32 1
            # "when selecting a value\nbigger than possible\nnos or nob, a dummy \nvalue \"1\" is chosen\n\nTODO:\ninsert error handling\nwith lower values than 1"
            # "display"
            n147 = event-data() -> ()  [unwired: 1 in, 6 out]
            n148 = global read "Globals.vi" "boards"() -> (w158:u32)
            n149 = global read "Globals.vi" "nob"() -> (w147:u32)
            n150 = global read "Globals.vi" "nos"() -> (w154:u32)
            n151 = Greater Or Equal?(x=w147, y="block") -> (x >= y?=w150:bool)
            n152 = Greater Or Equal?(x=w154, y="sample") -> (x >= y?=w153:bool)
            n153 = global read "Globals.vi" "PIXEL"() -> (w144:u32)
            n154 = case shown="False" w150 {
              tunnel: [u32 1 w163] -> w149
              tunnel: "block" -> [_ w163]
              frame False {
                n155 = call "Display Message to User"() -> ()  [unwired: 10 in, 2 out]
              }
              frame True {
              }
            }
            n156 = case shown="False" w153 {
              tunnel: [u32 1 w165] -> w152
              tunnel: "sample" -> [_ w165]
              frame False {
                n157 = call "Display Message to User2"() -> ()  [unwired: 10 in, 2 out]
              }
              frame True {
              }
            }
            n158 = To Long Integer(number=w144) -> (32bit integer=w145:i32)
            n159 = Initialize Array(u16 100, w145) -> (w161:u16[])
            n160 = Subtract(x=w152, y=w155) -> (x-y=w157:u32)
            n161 = Subtract(x=w149, y=w155) -> (x-y=w156:u32)
            n162 = case shown="2" w158 {
              selector: w158 -> [_ w170]
              tunnel: w157 -> [_ w171]
              tunnel: w156 -> [_ w168]
              frame 0, Default {
              }
              frame 2 {
                n163 = global read "Globals.vi" "PIXEL"() -> (w166:u32)
                n164 = To Long Integer(number=w166) -> (32bit integer=w167:i32)
                n165 = Initialize Array(u16 100, w167) -> (w173:u16[])
                n166 = call "ReturnFrame.vi"("Data Values In"=w173, "curr_nob"=w168, "curr_nos"=w171, "Drv"=w170) -> ("Data Values Out"=→"Signalverlaufgraph 2":u16[])  [unwired: 1 in]
              }
            }
            n167 = call "ReturnFrame.vi"("Data Values In"=w161, "curr_nob"=w156, "curr_nos"=w157, "Drv"=u32 1) -> ("Data Values Out"=→"Signalverlaufgraph":u16[])  [unwired: 1 in]
          }
          event "channel quick select (in hex)": Value Change {
            # "channel and camera select via quick select"
            n168 = event-data() -> ()  [unwired: 1 in, 6 out]
            n169 = flat-sequence {
              frame #0 {
                n170 = Number To Boolean Array(number="channel quick select (in hex)") -> (Boolean array=w221:bool[])
                n171 = Number To Boolean Array(number="channel quick select (in hex)") -> (Boolean array=w223:bool[])
                n172 = Number To Boolean Array(number="channel quick select (in hex)") -> (Boolean array=w213:bool[])
                n173 = Number To Boolean Array(number="channel quick select (in hex)") -> (Boolean array=w219:bool[])
                n174 = Number To Boolean Array(number="channel quick select (in hex)") -> (Boolean array=w215:bool[])
                n175 = Number To Boolean Array(number="channel quick select (in hex)") -> (Boolean array=w217:bool[])
                n176 = Number To Boolean Array(number="channel quick select (in hex)") -> (Boolean array=w209:bool[])
                n177 = Number To Boolean Array(number="channel quick select (in hex)") -> (Boolean array=w211:bool[])
                n178 = Index Array(array=w221, index=6) -> (element=w195:bool)
                n179 = Index Array(array=w223, index=7) -> (element=w194:bool)
                n180 = Index Array(array=w213, index=1) -> (element=w207:bool)
                n181 = Index Array(array=w219, index=5) -> (element=w199:bool)
                n182 = Index Array(array=w215, index=3) -> (element=w204:bool)
                n183 = Index Array(array=w217, index=4) -> (element=w200:bool)
                n184 = Index Array(array=w209, index=0) -> (element=w208:bool)
                n185 = Index Array(array=w211, index=2) -> (element=w205:bool)
                n186 = Or(x=w195, y=w194) -> (x .or. y?=w196:bool)
                n187 = Or(x=w200, y=w199) -> (x .or. y?=w198:bool)
                n188 = Or(x=w208, y=w207) -> (x .or. y?=w206:bool)
                n189 = Or(x=w205, y=w204) -> (x .or. y?=w203:bool)
                n190 = Build Array(w206) -> (w202:bool[])
                n191 = Build Array (concatenate)(w202, w203) -> (w201:bool[])
                n192 = Build Array (concatenate)(w201, w198) -> (w197:bool[])
                n193 = Build Array (concatenate)(w197, w196) -> (w193:bool[])
                n194 = property on="CHA 4" class="Bool (strict)"("Value"=w195) -> ()  [unwired: 2 in, 2 out]
                n195 = property on="CHB 4" class="Bool (strict)"("Value"=w194) -> ()  [unwired: 2 in, 2 out]
                n196 = property on="CHB 1" class="Bool (strict)"("Value"=w207) -> ()  [unwired: 2 in, 2 out]
                n197 = property on="CHB 3" class="Bool (strict)"("Value"=w199) -> ()  [unwired: 2 in, 2 out]
                n198 = property on="CHB 2" class="Bool (strict)"("Value"=w204) -> ()  [unwired: 2 in, 2 out]
                n199 = property on="CHA 3" class="Bool (strict)"("Value"=w200) -> ()  [unwired: 2 in, 2 out]
                n200 = property on="CHA 1" class="Bool (strict)"("Value"=w208) -> ()  [unwired: 2 in, 2 out]
                n201 = property on="CHA 2" class="Bool (strict)"("Value"=w205) -> ()  [unwired: 2 in, 2 out]
                n202 = Number To Boolean Array(number="channel quick select (in hex)") -> (Boolean array=w237:bool[])
                n203 = Number To Boolean Array(number="channel quick select (in hex)") -> (Boolean array=w239:bool[])
                n204 = Number To Boolean Array(number="channel quick select (in hex)") -> (Boolean array=w229:bool[])
                n205 = Number To Boolean Array(number="channel quick select (in hex)") -> (Boolean array=w235:bool[])
                n206 = Number To Boolean Array(number="channel quick select (in hex)") -> (Boolean array=w231:bool[])
                n207 = Number To Boolean Array(number="channel quick select (in hex)") -> (Boolean array=w233:bool[])
                n208 = Number To Boolean Array(number="channel quick select (in hex)") -> (Boolean array=w225:bool[])
                n209 = Number To Boolean Array(number="channel quick select (in hex)") -> (Boolean array=w227:bool[])
                n210 = Index Array(array=w237, index=14) -> (element=w179:bool)
                n211 = Index Array(array=w239, index=15) -> (element=w178:bool)
                n212 = Index Array(array=w229, index=9) -> (element=w190:bool)
                n213 = Index Array(array=w235, index=13) -> (element=w180:bool)
                n214 = Index Array(array=w231, index=11) -> (element=w188:bool)
                n215 = Index Array(array=w233, index=12) -> (element=w181:bool)
                n216 = Index Array(array=w225, index=8) -> (element=w191:bool)
                n217 = Index Array(array=w227, index=10) -> (element=w189:bool)
                n218 = Or(x=w191, y=w190) -> (x .or. y?=w192:bool)
                n219 = Or(x=w181, y=w180) -> (x .or. y?=w184:bool)
                n220 = Or(x=w189, y=w188) -> (x .or. y?=w186:bool)
                n221 = Or(x=w179, y=w178) -> (x .or. y?=w182:bool)
                n222 = Build Array (concatenate)(w193, w192) -> (w187:bool[])
                n223 = Build Array (concatenate)(w187, w186) -> (w185:bool[])
                n224 = Build Array (concatenate)(w185, w184) -> (w183:bool[])
                n225 = Build Array (concatenate)(w183, w182) -> (w174:bool[])
                n226 = property on="CHA 8" class="Bool (strict)"("Value"=w179) -> ()  [unwired: 2 in, 2 out]
                n227 = property on="CHB 8" class="Bool (strict)"("Value"=w178) -> ()  [unwired: 2 in, 2 out]
                n228 = property on="CHB 5" class="Bool (strict)"("Value"=w190) -> ()  [unwired: 2 in, 2 out]
                n229 = property on="CHB 7" class="Bool (strict)"("Value"=w180) -> ()  [unwired: 2 in, 2 out]
                n230 = property on="CHB 6" class="Bool (strict)"("Value"=w188) -> ()  [unwired: 2 in, 2 out]
                n231 = property on="CHA 7" class="Bool (strict)"("Value"=w181) -> ()  [unwired: 2 in, 2 out]
                n232 = property on="CHA 5" class="Bool (strict)"("Value"=w191) -> ()  [unwired: 2 in, 2 out]
                n233 = property on="CHA 6" class="Bool (strict)"("Value"=w189) -> ()  [unwired: 2 in, 2 out]
                n234 = Number To Boolean Array(number="channel quick select (in hex)") -> (Boolean array=w247:bool[])
                n235 = global read "Globals.vi" "maddr of CC"() -> (w241:u8)
                n236 = Boolean To (0,1)(Boolean=w247) -> (0, 1=w243:i16[])
                n237 = global read "Globals.vi" "reg_addr-CH_select"() -> (w242:u8)
                n238 = Boolean To (0,1)(Boolean=w174) -> (0, 1=w177:i16[])
                n239 = Add Array Elements(numeric array=w243) -> (sum=w245:i16)
                n240 = Add Array Elements(numeric array=w177) -> (sum=w176:i16)
                n241 = To Unsigned Byte Integer(number=w245) -> (unsigned 8bit integer=w244:u8)
                n242 = To Unsigned Byte Integer(number=w176) -> (unsigned 8bit integer=w175:u8)
                n243 = call "SendFLCam.vi"("madr"=w241, "data"="channel quick select (in hex)", "adadr"=w242) -> ()
                n244 = global write "Globals.vi" "devices_amount"(w175) -> ()
                n245 = global write "Globals.vi" "cams_amount"(w244) -> ()
              }
              frame #1 {
                # "refresh nos for triggering MB calc"
                n246 = global read "Globals.vi" "devices_amount"() -> (w249:u8)
                n247 = global read "Globals.vi" "cams_amount"() -> (w250:u8)
                n248 = property on="no.of blocks (nob)\npress enter" class="DigNum (strict)"() -> ("Value"=w248:u32)  [unwired: 2 in, 2 out]
                n249 = property on="amount of cams" class="DigNum (strict)"("Value"=w250) -> ()  [unwired: 2 in, 2 out]
                n250 = property on="no.of blocks (nob)\npress enter" class="DigNum (strict)"("Val(Sgnl)"=w248) -> ()  [unwired: 2 in, 2 out]
                n251 = property on="amount of devices" class="DigNum (strict)"("Value"=w249) -> ()  [unwired: 2 in, 2 out]
              }
            }
          }
          event "CHA 1", "CHB 1", "CHA 2", "CHB 2", "CHA 3", "CHB 3", "CHA 4", "CHB 4", "CHA 5", "CHB 5", "CHA 6", "CHB 6", "CHA 7", "CHB 7", "CHA 8", "CHB 8": Value Change {
            # "channel and camera select via switches"
            n252 = event-data() -> ()  [unwired: 1 in, 6 out]
            n253 = flat-sequence {
              frame #0 {
                n254 = Or(x="CHB 4", y="CHA 4") -> (x .or. y?=w263:bool)
                n255 = Or(x="CHB 3", y="CHA 3") -> (x .or. y?=w265:bool)
                n256 = Build Array("CHA 1") -> (w290:bool[])
                n257 = Build Array (concatenate)(w290, "CHB 1") -> (w291:bool[])
                n258 = Or(x="CHB 2", y="CHA 2") -> (x .or. y?=w267:bool)
                n259 = Build Array (concatenate)(w291, "CHA 2") -> (w292:bool[])
                n260 = Build Array (concatenate)(w292, "CHB 2") -> (w293:bool[])
                n261 = Build Array (concatenate)(w293, "CHA 3") -> (w294:bool[])
                n262 = Build Array (concatenate)(w294, "CHB 3") -> (w295:bool[])
                n263 = Build Array (concatenate)(w295, "CHA 4") -> (w296:bool[])
                n264 = Build Array (concatenate)(w296, "CHB 4") -> (w297:bool[])
                n265 = Or(x="CHA 1", y="CHB 1") -> (x .or. y?=w269:bool)
                n266 = Build Array(w269) -> (w268:bool[])
                n267 = Build Array (concatenate)(w268, w267) -> (w266:bool[])
                n268 = Build Array (concatenate)(w266, w265) -> (w264:bool[])
                n269 = Build Array (concatenate)(w264, w263) -> (w262:bool[])
                n270 = Build Array (concatenate)(w297, "CHA 5") -> (w298:bool[])
                n271 = Build Array (concatenate)(w298, "CHB 5") -> (w299:bool[])
                n272 = Build Array (concatenate)(w299, "CHA 6") -> (w300:bool[])
                n273 = Build Array (concatenate)(w300, "CHB 6") -> (w301:bool[])
                n274 = Build Array (concatenate)(w301, "CHA 7") -> (w302:bool[])
                n275 = Build Array (concatenate)(w302, "CHB 7") -> (w303:bool[])
                n276 = Build Array (concatenate)(w303, "CHA 8") -> (w304:bool[])
                n277 = Build Array (concatenate)(w304, "CHB 8") -> (w289:bool[])
                n278 = Or(x="CHA 5", y="CHB 5") -> (x .or. y?=w261:bool)
                n279 = Or(x="CHB 6", y="CHA 6") -> (x .or. y?=w259:bool)
                n280 = Or(x="CHA 7", y="CHB 7") -> (x .or. y?=w257:bool)
                n281 = Or(x="CHA 8", y="CHB 8") -> (x .or. y?=w255:bool)
                n282 = Boolean To (0,1)(Boolean=w289) -> (0, 1=w288:i16[])
                n283 = Boolean Array To Number(Boolean array=w289) -> (number=w305:u32)
                n284 = Build Array (concatenate)(w262, w261) -> (w260:bool[])
                n285 = Build Array (concatenate)(w260, w259) -> (w258:bool[])
                n286 = Build Array (concatenate)(w258, w257) -> (w256:bool[])
                n287 = Build Array (concatenate)(w256, w255) -> (w254:bool[])
                n288 = Add Array Elements(numeric array=w288) -> (sum=w286:i16)
                n289 = To Unsigned Word Integer(number=w305) -> (unsigned 16bit integer=w306:u16)
                n290 = To Unsigned Byte Integer(number=w286) -> (unsigned 8bit integer=w287:u8)
                n291 = Boolean To (0,1)(Boolean=w254) -> (0, 1=w253:i16[])
                n292 = Add Array Elements(numeric array=w253) -> (sum=w252:i16)
                n293 = global write "Globals.vi" "cams_amount"(w287) -> ()
                n294 = property on="channel quick select (in hex)" class="DigNum (strict)"("Value"=w306) -> ()  [unwired: 2 in, 2 out]
                n295 = To Unsigned Byte Integer(number=w252) -> (unsigned 8bit integer=w251:u8)
                n296 = global write "Globals.vi" "devices_amount"(w251) -> ()
              }
              frame #1 {
                # "refresh nos for triggering MB calc"
                n297 = global read "Globals.vi" "devices_amount"() -> (→"amount of devices":u8)
                n298 = global read "Globals.vi" "cams_amount"() -> (→"amount of cams":u8)
                n299 = global read "Globals.vi" "maddr of CC"() -> (w310:u8)
                n300 = global read "Globals.vi" "reg_addr-CH_select"() -> (w311:u8)
                n301 = property on="channel quick select (in hex)" class="DigNum (strict)"() -> ("Value"=w312:u16)  [unwired: 2 in, 2 out]
                n302 = call "SendFLCam.vi"("madr"=w310, "data"=w312, "adadr"=w311) -> ()
                n303 = property on="no.of samples (nos)" class="DigNum (strict)"() -> ("Value"=w307:u32)  [unwired: 2 in, 2 out]
                n304 = property on="no.of samples (nos)" class="DigNum (strict)"("Val(Sgnl)"=w307) -> ()  [unwired: 2 in, 2 out]
              }
            }
          }
          event "no.of samples (nos)", "no.of blocks (nob)\npress enter", "exposuretime[ms]": Value Change {
            # "calculation of MB RAM an SEC and setting scale max"
            # "MB"
            # "ushort"
            n305 = event-data() -> ()  [unwired: 1 in, 7 out]
            n306 = global read "Globals.vi" "PIXEL"() -> (w338:u32)
            n307 = Multiply(x="no.of samples (nos)", y=w338) -> (x*y=w336:u32)
            n308 = Multiply(x=w336, y=u32 2) -> (x*y=w316:u32)
            n309 = global read "Globals.vi" "boards"() -> (w337:u32)
            n310 = global read "Globals.vi" "cams_amount"() -> (w315:u8)
            n311 = global read "Globals.vi" "nos"() -> (w320:u32)
            n312 = global read "Globals.vi" "nob"() -> (w318:u32)
            n313 = To Unsigned Long Integer(number=w315) -> (unsigned 32bit integer=w314:u32)
            n314 = Multiply(x=w314, y=w316) -> (x*y=w313:u32)
            n315 = Multiply(x=w313, y=w337) -> (x*y=w326:u32)
            n316 = To Double Precision Float(number=w326) -> (double precision float=w325:dbl)
            n317 = To Double Precision Float(number=w320) -> (double precision float=w319:dbl)
            n318 = Divide(x=w325, y=1048576.0) -> (x/y=w328:dbl)
            n319 = To Double Precision Float(number=w318) -> (double precision float=w317:dbl)
            n320 = To Double Precision Float(number="no.of blocks (nob)\npress enter") -> (double precision float=w323:dbl)
            n321 = property on="sample" class="Slide (strict)"("Scale.Maximum"=w319) -> ()  [unwired: 2 in, 2 out]
            n322 = property on="block" class="Slide (strict)"("Scale.Maximum"=w317) -> ()  [unwired: 2 in, 2 out]
            n323 = Multiply(x=w328, y=w323) -> (x*y=→"MB RAM":dbl)
            n324 = global write "Globals.vi" "nos"("no.of samples (nos)") -> ()
            n325 = Multiply(x="no.of samples (nos)", y="no.of blocks (nob)\npress enter") -> (x*y=w321:u32)
            n326 = global write "Globals.vi" "nob"("no.of blocks (nob)\npress enter") -> ()
            n327 = To Double Precision Float(number=w321) -> (double precision float=w322:dbl)
            n328 = global write "Globals.vi" "exp time"("exposuretime[ms]") -> ()
            n329 = Multiply(x="exposuretime[ms]", y=w322) -> (x*y=w334:dbl)
            n330 = Divide(x=w334, y=1000.0) -> (x/y=→"SEC":dbl)
          }
          event "stop all": Value Change {
            # "exit"
            n331 = event-data() -> ()  [unwired: 1 in, 6 out]
            n332 = stacked-sequence {
              tunnel: [_ TRUE] -> w339
              frame #0 {
                n333 = call "FFStop.vi"() -> ()  [unwired: 1 in]
              }
              frame #1 {
                # "do not omit, or next call of driver will go wrong."
                n334 = call "Exit.vi"() -> ()  [unwired: 1 in]
              }
            }
          }
          event "rms_pixel": Value Change {
            # "one array with all values (except first 10)\nat index Pixel from all blocks"
            n335 = event-data() -> ()  [unwired: 1 in, 6 out]
            n336 = global read "Globals.vi" "nos"() -> (w345:u32)
            n337 = global read "Globals.vi" "nob"() -> (w346:u32)
            n338 = for {
              N: w346 -> [_]
              tunnel: w345 -> [w347]
              tunnel: [w349] -> w342 mode=concatenating
              i -> [w353]
              # "delete first 10 values"
              # "array of all values\nat index Pixel"
              n339 = To Long Integer(number=w347) -> (32bit integer=w348:i32)
              n340 = for {
                N: w348 -> [_]
                tunnel: w353 -> [w358]
                tunnel: [w362] -> w350 mode=indexing
                i -> [w360]
                # "use only value at index \"Pixel\""
                # "init array of size PIXEL\nwith value 100"
                n341 = global read "Globals.vi" "PIXEL"() -> (w354:u32)
                n342 = To Long Integer(number=w354) -> (32bit integer=w355:i32)
                n343 = To Unsigned Long Integer(number=w358) -> (unsigned 32bit integer=w359:u32)
                n344 = To Unsigned Long Integer(number=w360) -> (unsigned 32bit integer=w361:u32)
                n345 = Initialize Array(u16 100, w355) -> (w364:u16[])
                n346 = call "ReturnFrame.vi"("Data Values In"=w364, "curr_nob"=w359, "curr_nos"=w361, "Drv"=u32 1) -> ("Data Values Out"=w363:u16[])  [unwired: 1 in]
                n347 = To Long Integer(number="rms_pixel") -> (32bit integer=w356:i32)
                n348 = Index Array(array=w363, index=w356) -> (element=w362:u16)
              }
              n349 = Delete From Array(array=w350, length=10, index=0) -> (array with subset deleted=w349:u16[])  [unwired: 1 out]
            }
            n350 = To Double Precision Float(number=w342) -> (double precision float=w341:dbl[])
            n351 = call <vilib>:"Std Deviation and Variance.vi"("X"=w341) -> ("mean"=→"mean":dbl, "standard deviation"=→"tRMS":dbl)  [unwired: 1 in, 1 out]
          }
        }
      }
    }
  }
  n352 = property on="sample" class="Slide (strict)"("DisabledEnum"=w1) -> ()  [unwired: 2 in, 2 out]
  n353 = property on="start" class="Bool (strict)"("DisabledEnum"=w1) -> ()  [unwired: 2 in, 2 out]
  n354 = property on="block" class="Slide (strict)"("DisabledEnum"=w1) -> ()  [unwired: 2 in, 2 out]
